vi "Configure Channel (DI Delta).vi"(0 "VISA resource name":refnum<visa-resource-name>, 1 "Reference Channel (0001)":string="0001", 5 "Channel (0001)":string="0001", 7 "Enable Channel (True)":bool=TRUE, 9 "Span":T1={"Lower Span (0)"=0, "Upper Span (1)"=1} {"Upper Span (1)" min=-99999 max=99999 step=1; "Lower Span (0)" min=-99999 max=99999 step=1}, 11 "error in (no error)":errorcluster) -> (4 "VISA resource name out":refnum<visa-resource-name>, 6 "Channel":string, 15 "error out":errorcluster)   [LabVIEW 2020, in "Yokogawa GX Series.lvlib"]
doc: "Sets the input range of DI channels.\n\nCommand: SRangeDI"
uses:
  <instrlib>/Yokogawa GX Series/Yokogawa GX Series.lvlib
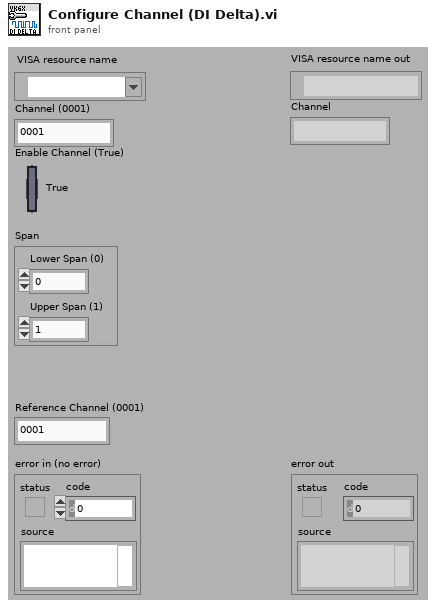
[diagram p1: front panel]
types:
  T1 = cluster{"Lower Span (0)":i32, "Upper Span (1)":i32}
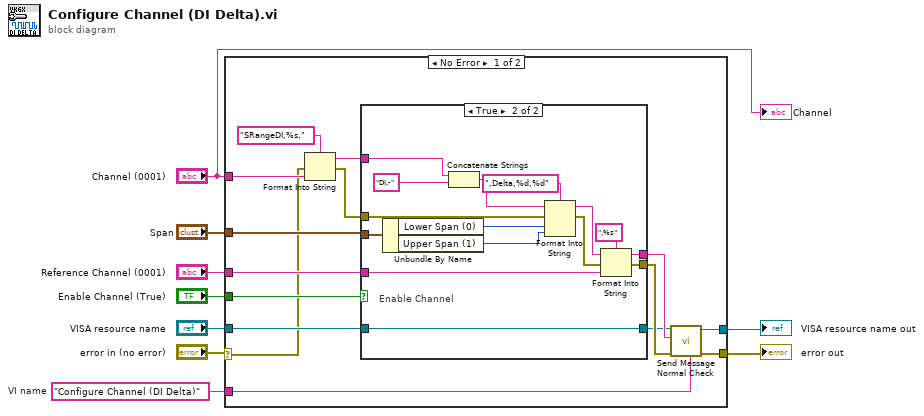
[diagram p0: block diagram]
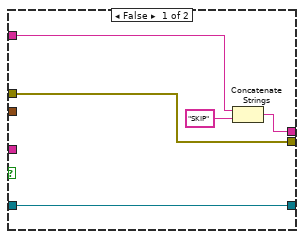
[diagram p2: hidden frame]
diagram:
  w7 = "Configure Channel (DI Delta)"  # VI name
  n1 = case shown="No Error" "error in (no error)" {
    selector: "error in (no error)" -> [w10 w45]
    tunnel: "Reference Channel (0001)" -> [w21 _]
    tunnel: "Enable Channel (True)" -> [w20 _]
    tunnel: w7 -> [w17 _]
    tunnel: [w16 w46] -> w6
    tunnel: [w15 w45] -> w5
    tunnel: "Channel (0001)" -> [w14 _]
    tunnel: "VISA resource name" -> [w13 w46]
    tunnel: "Span" -> [w11 _]
    frame No Error {
      n2 = Format Into String(format string="SRangeDI,%s,", error in=w10, w14) -> (resulting string=w22:string, error out=w23:errorcluster)  [unwired: 1 in]
      n3 = case shown="True" w20 {
        tunnel: w23 -> [w26 w43]
        tunnel: w22 -> [w27 w42]
        tunnel: w21 -> [_ w41]
        tunnel: [w26 w37] -> w19
        tunnel: [w28 w36] -> w18
        tunnel: w11 -> [_ w34]
        tunnel: w13 -> [w25 w30]
        tunnel: [w25 w30] -> w12
        frame False {
          n4 = Concatenate Strings(w27, "SKIP") -> (w28:string)
        }
        frame True {
          # "Enable Channel"
          n5 = Unbundle By Name(w34) -> ("Lower Span (0)"=w32:i32, "Upper Span (1)"=w31:i32)
          n6 = Concatenate Strings(w42, "DI,-") -> (w33:string)
          n7 = Format Into String(format string=",Delta,%d,%d", initial string=w33, error in=w43, w32, w31) -> (resulting string=w38:string, error out=w39:errorcluster)
          n8 = Format Into String(format string=",%s", initial string=w38, error in=w39, w41) -> (resulting string=w36:string, error out=w37:errorcluster)
        }
      }
      n9 = call <instrlib>:"Send Message Normal Check.vi"("Source (\"\")"=w17, "error in (no error)"=w19, "Send Message (\"\")"=w18, "VISA resource name"=w12) -> ("error out"=w15:errorcluster, "VISA resource name out"=w16:refnum<visa-resource-name>)  [unwired: 2 in, 4 out]
    }
    frame Error {
    }
  }
  "error out" <- w5
  "VISA resource name out" <- w6
  "Channel" <- "Channel (0001)"
